vi "writeWaitForRx.vi"(8 "error in (no error)":errorcluster, 10 "Timeout(us)":u32, 11 "ModbusBuffer in":refnum<class "ModbusBuffer.lvclass">) -> (0 "error out":errorcluster, 3 "ModbusBuffer out":refnum<class "ModbusBuffer.lvclass">)   [LabVIEW 2016, in "RTModbus.lvlib" / "ModbusBuffer.lvclass"]
uses:
  ModbusBuffer.lvclass
  ModbusBuffer.lvclass/ModbusBuffer.ctl
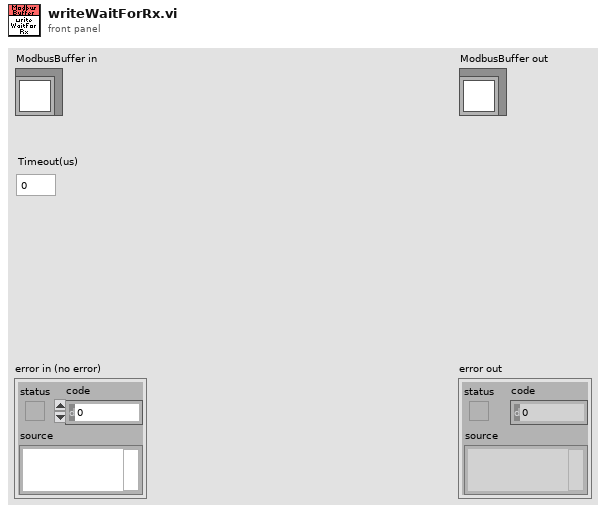
[diagram p1: front panel]
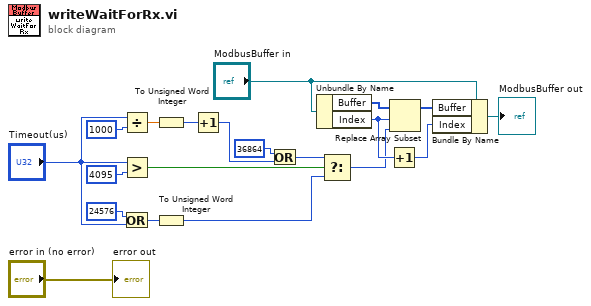
[diagram p0: block diagram]
diagram:
  n1 = Divide(x="Timeout(us)", y=u32 1000) -> (x/y=w18:dbl)
  n2 = Greater?(x="Timeout(us)", y=u32 4095) -> (0:w17:bool)
  n3 = Or(x=u16 24576, y="Timeout(us)") -> (x .or. y?=w2:u32)
  n4 = To Unsigned Word Integer(number=w18) -> (unsigned 16bit integer=w16:u16)
  n5 = To Unsigned Word Integer(number=w2) -> (unsigned 16bit integer=w1:u16)
  n6 = Increment(x=w16) -> (x+1=w6:u16)
  n7 = Or(x=u16 36864, y=w6) -> (x .or. y?=w4:u16)
  n8 = Unbundle By Name("ModbusBuffer in") -> ("Buffer"=w15:u16[], "Index"=w11:i32)
  n9 = Select(t=w4, s=w17, f=w1) -> (s? t:f=w7:u16)
  n10 = Increment(x=w11) -> (x+1=w10:i32)
  n11 = Replace Array Subset(array=w15, new element=w7, index=w11) -> (w12:u16[])
  n12 = Bundle By Name(cluster="ModbusBuffer in", "Buffer"=w12, "Index"=w10) -> (→"ModbusBuffer out":refnum<class "ModbusBuffer.lvclass">)
  "error out" <- "error in (no error)"
